vi "SubVI_HandleFileChanges.vi"(0 "File Refnum in":refnum<k34>, 1 "Independent?":bool, 3 "notifier in":refnum<notifier>, 5 "Numeric":i32, 7 "Sava data tured on or off?":bool, 9 "Save Data TDMS":bool, 11 "error in (no error)":errorcluster, 12 "File Info Changed?":bool, 13 "VI name":string="Sensors_DAQ") -> (4 "File Refnum out":refnum<k34>, 15 "error out":errorcluster)   [LabVIEW 2018]
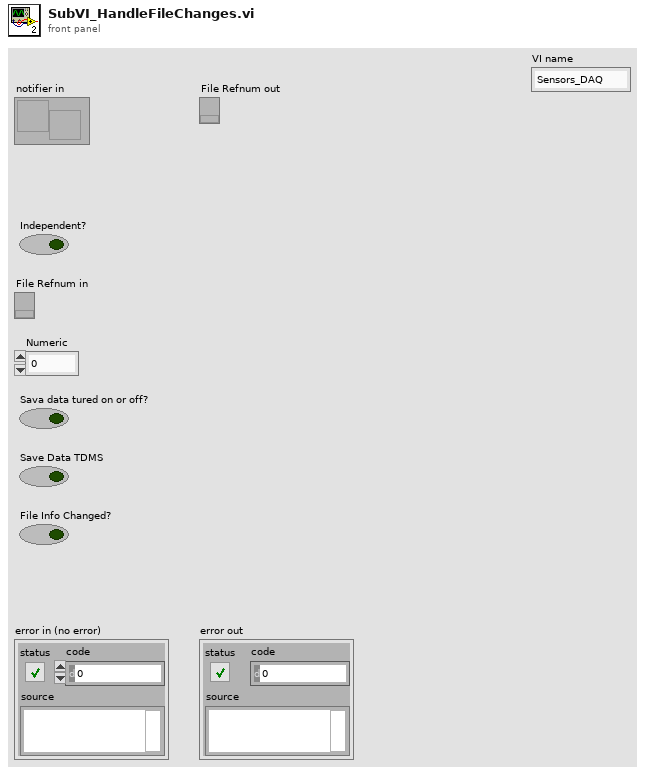
[diagram p1: front panel]
types:
  T1 = enum16{"open", "open or create", "create or replace", "create", "open (read-only)"}
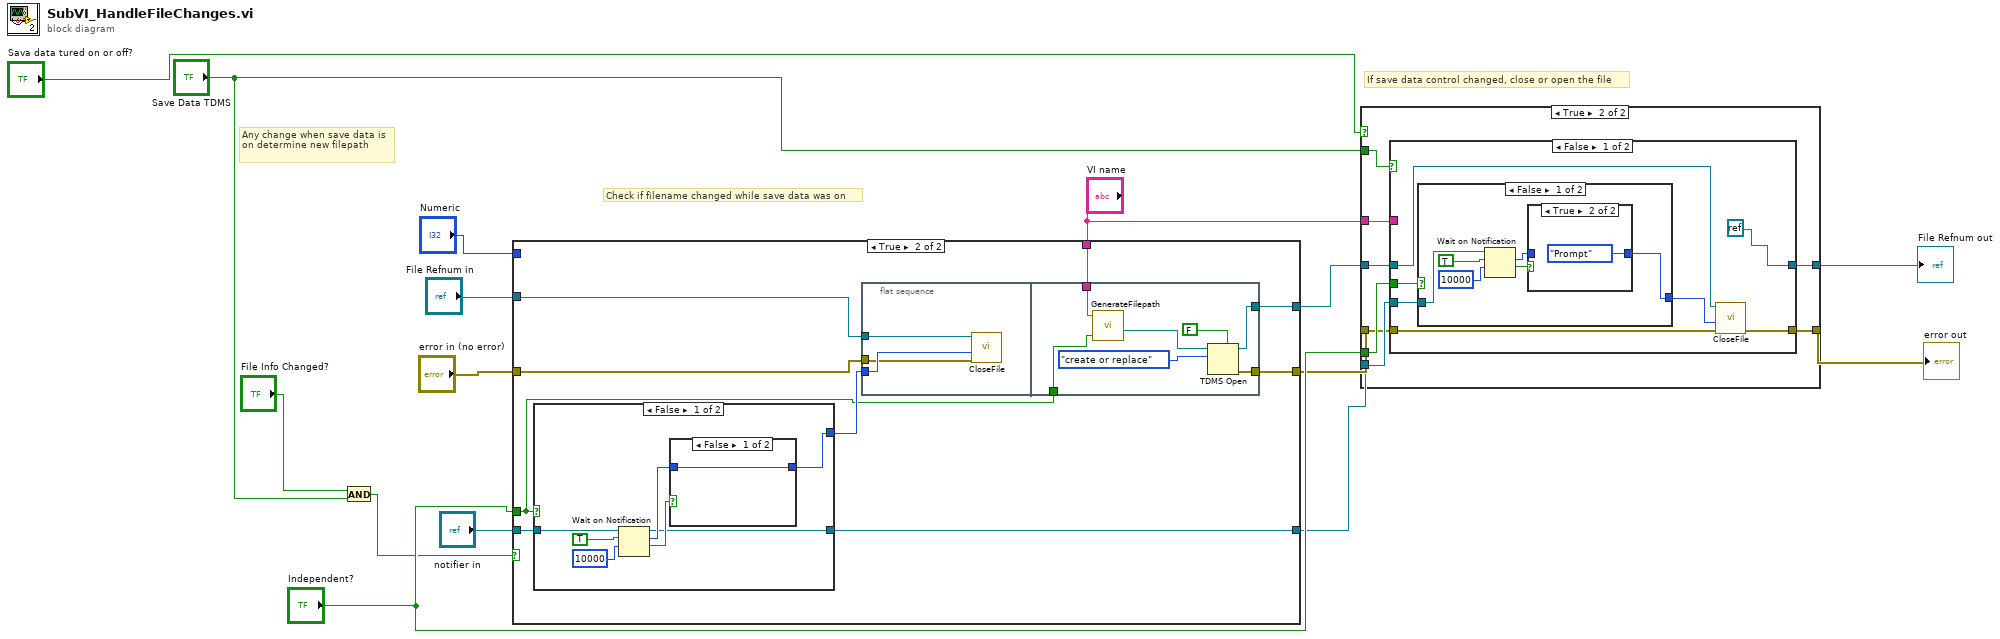
[diagram p0: block diagram]
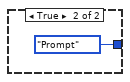
[diagram p4: hidden frame]
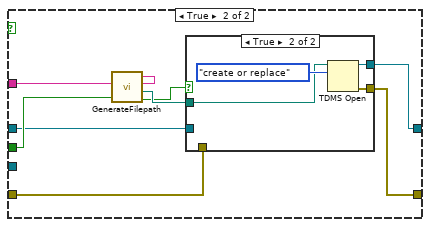
[diagram p5: hidden frame]
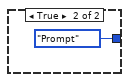
[diagram p8: hidden frame]
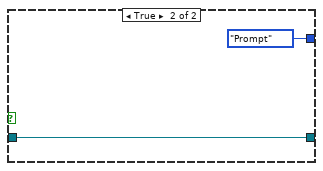
[diagram p9: hidden frame]
diagram:
  # "If save data control changed, close or open the file"
  # "Any change when save data is on determine new filepath"
  # "Check if filename changed while save data was on"
  n1 = And(x="File Info Changed?", y="Save Data TDMS") -> (x .and. y?=w1:bool)
  n2 = case shown="True" w1 {
    tunnel: "notifier in" -> [w18 w27]
    tunnel: "Numeric" -> [_ _]
    tunnel: "Independent?" -> [_ w19]
    tunnel: [w18 w26] -> w7
    tunnel: "File Refnum in" -> [w16 w24]
    tunnel: "error in (no error)" -> [w17 w23]
    tunnel: [w16 w22] -> w12
    tunnel: [w17 w21] -> w13
    tunnel: "VI name" -> [_ w20]
    frame False {
    }
    frame True {
      n3 = case shown="False" w19 {
        tunnel: [w39 enum16{"Prompt", "Keep", "Archive", "Trash"}."Prompt" ("NewVal")] -> w25
        tunnel: w27 -> [w44 w47]
        tunnel: [w38 w47] -> w26
        frame False {
          n4 = Wait on Notification(notifier=w44, ignore previous (F)=TRUE, timeout in ms (-1)=10000) -> (notifier out=w38:refnum<notifier>, notification=w40:enum16{"Prompt", "Keep", "Archive", "Trash"}, timed out?=w41:bool)  [unwired: 1 in, 1 out]
          n5 = case shown="False" w41 {
            tunnel: w40 -> [w45 _]
            tunnel: [w45 enum16{"Prompt", "Keep", "Archive", "Trash"}."Prompt" ("Action")] -> w39
            frame False {
            }
            frame True {
            }
          }
        }
        frame True {
        }
      }
      n6 = flat-sequence {
        tunnel: w25 -> [w30]
        tunnel: w24 -> [w29]
        tunnel: w23 -> [w28]
        tunnel: [w35] -> w22
        tunnel: [w34] -> w21
        tunnel: w20 -> [w33]
        tunnel: w19 -> [w32]
        frame #0 {
          n7 = call "CloseFile.vi"("error in (no error)"=w28, "Action"=w30, "Refnum in"=w29) -> ()  [unwired: 6 in, 3 out]
        }
        frame #1 {
          n8 = call "GenerateFilepath.vi"("Instrument"=w33, "Check for file?"=w32) -> ("File Path Out"=w31:path)  [unwired: 3 in, 1 out]
          n9 = TDMS Open(5:FALSE ("create index file? (T)"), 10:T1."create or replace" ("operation (0:open)"), 11:w31) -> (0:w34:errorcluster, 3:w35:refnum<k34>)  [unwired: 4 in]
        }
      }
    }
  }
  n10 = case shown="True" "Sava data tured on or off?" {
    tunnel: "Independent?" -> [_ w58]
    tunnel: w7 -> [_ w57]
    tunnel: [w50 w56] -> w10
    tunnel: [w49 w55] -> w11
    tunnel: w12 -> [w50 w54]
    tunnel: w13 -> [w49 w53]
    tunnel: "Save Data TDMS" -> [_ w52]
    tunnel: "VI name" -> [_ w51]
    frame False {
    }
    frame True {
      n11 = case shown="False" w52 {
        tunnel: w58 -> [w64 w79]
        tunnel: w57 -> [w63 _]
        tunnel: w54 -> [w62 w76]
        tunnel: w53 -> [w61 w75]
        tunnel: [refnum<k0> refnum w82] -> w56
        tunnel: [w60 w81] -> w55
        tunnel: w51 -> [_ w80]
        frame False {
          n12 = case shown="False" w64 {
            tunnel: [w66 enum16{"Prompt", "Keep", "Archive", "Trash"}."Prompt" ("NewVal")] -> w65
            tunnel: w63 -> [w70 _]
            frame False {
              n13 = Wait on Notification(notifier=w70, ignore previous (F)=TRUE, timeout in ms (-1)=10000) -> (notification=w67:enum16{"Prompt", "Keep", "Archive", "Trash"}, timed out?=w68:bool)  [unwired: 1 in, 2 out]
              n14 = case shown="True" w68 {
                tunnel: w67 -> [w72 _]
                tunnel: [w72 enum16{"Prompt", "Keep", "Archive", "Trash"}."Prompt" ("Action")] -> w66
                frame False {
                }
                frame True {
                }
              }
            }
            frame True {
            }
          }
          n15 = call "CloseFile.vi"("error in (no error)"=w61, "Action"=w65, "Refnum in"=w62) -> ("error out"=w60:errorcluster)  [unwired: 6 in, 2 out]
        }
        frame True {
          n16 = call "GenerateFilepath.vi"("Instrument"=w80, "Check for file?"=w79) -> ("File Path Out"=w78:path, "Create File?"=w77:bool)  [unwired: 3 in]
          n17 = case shown="True" w77 {
            tunnel: [w84 w87] -> w82
            tunnel: [w83 w86] -> w81
            tunnel: w78 -> [_ w85]
            tunnel: w76 -> [w84 _]
            tunnel: w75 -> [w83 _]
            frame False {
            }
            frame True {
              n18 = TDMS Open(10:T1."create or replace" ("operation (0:open)"), 11:w85) -> (0:w86:errorcluster, 3:w87:refnum<k34>)  [unwired: 5 in]
            }
          }
        }
      }
    }
  }
  "error out" <- w11
  "File Refnum out" <- w10
